vi "change pivot.vi"(6 "force recalc?":bool, 7 "Use bumper corners?":bool=TRUE, 8 "error in (no error)":errorcluster, 9 "new pivot center":T1 {"Y" format="%.4g"; "X" format="%.4g"}, 11 "select pivot point":T2) -> (0 "error out":errorcluster)   [LabVIEW 2023]
uses:
  ctrl defs/ctrl pivot select.ctl
  ctrl defs/ctrl XY coord.ctl
  ctrl defs/ctrl Wheel index.ctl
  Global odometry.vi
  Global INIT.vi
panel:
  in  "bumper (in)":dbl=3.5
  out "new pivot center 2":T1={"X"=-0.11812379110251395, "Y"=-0.5906189555125736} {"Y" format="%.4g"; "X" format="%.4g"}
  out "recalc mod polar":bool=TRUE
  out "output pivot center":T1={"X"=-0.11812379110251395, "Y"=-0.5906189555125736} {"Y" format="%.4g"; "X" format="%.4g"}
  out "Old pivot center":T1 {"Y" format="%.4g"; "X" format="%.4g"}
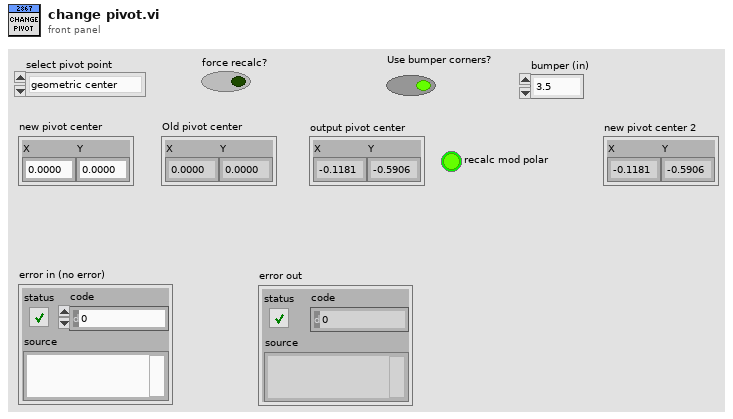
[diagram p1: front panel]
types:
  T1 = typedef "ctrl XY coord.ctl" = cluster{"X":dbl, "Y":dbl}
  T2 = typedef "ctrl pivot select.ctl" = enum16{"geometric center", "CG", "FL", "FR", "RR", "RL", "other"}
  T3 = typedef "ctrl robot swerve dims.ctl" = cluster{"width":dbl, "depth":dbl}
  T4 = cluster{"description":string, "wrt geom CTR":cluster{"delX":i8, "delY":i8}}[]
  T5 = typedef "ctrl swerve module.ctl" = cluster{"descr":string, "V":dbl, "POS":dbl, "target":dbl, "ABS":dbl, "from pivot to module":cluster{"R":dbl, "theta (deg)":dbl, "theta spin (deg)":dbl, "theta park (deg)":dbl}, "coord wrt geom CTR":cluster{"X":dbl, "Y":dbl}, "corner wt (lbm)":dbl}
  T6 = typedef "ctrl robot CG.ctl" = cluster{"mass (lbm)":dbl, "CG":T1, "Zcg":dbl}
  T7 = typedef "ctrl Wheel index.ctl" = enum16{"FR", "FL", "RL", "RR"}
  T8 = cluster{"description":string, "wrt geom CTR":cluster{"delX":i8, "delY":i8}}
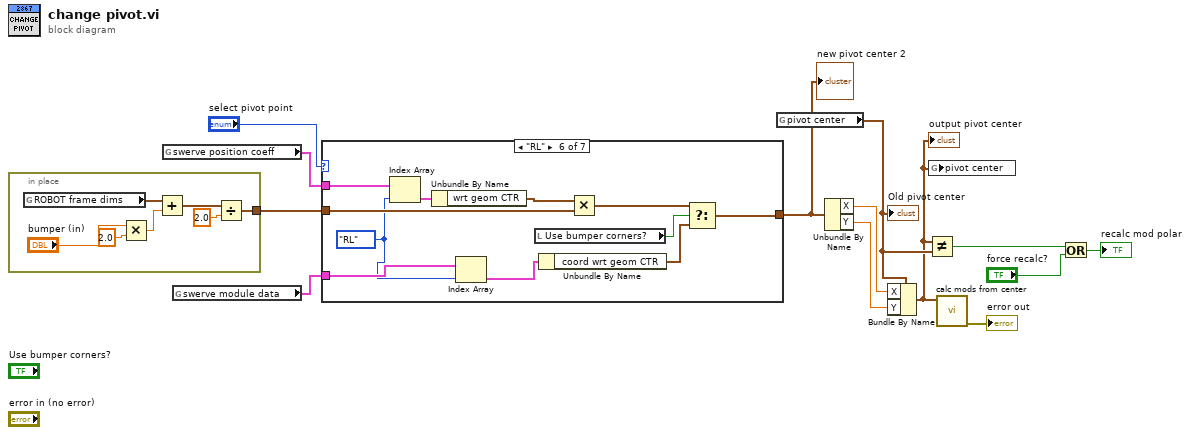
[diagram p0: block diagram]
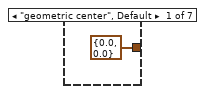
[diagram p2: hidden frame]
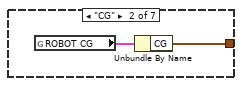
[diagram p3: hidden frame]
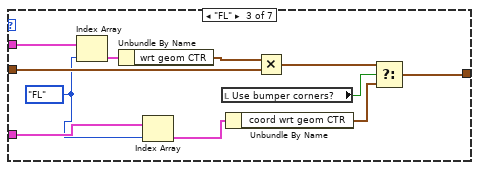
[diagram p4: hidden frame]
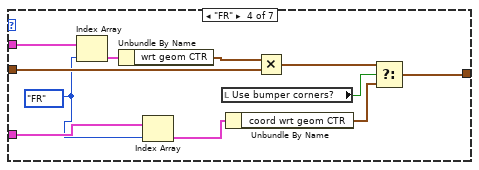
[diagram p5: hidden frame]
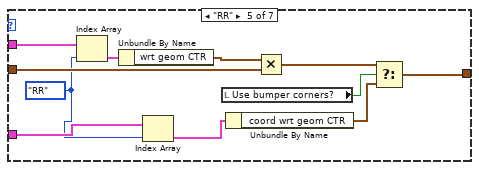
[diagram p6: hidden frame]
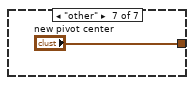
[diagram p7: hidden frame]
diagram:
  n1 = in-place {
    in-place-border: [w15] -> w2
    n2 = global read "Global INIT.vi" "ROBOT frame dims"() -> (w20:T3)
    n3 = Multiply(x="bumper (in)", y=2.0) -> (x*y=w19:dbl)
    n4 = Add(x=w20, y=w19) -> (x+y=w16:T3)
    n5 = Divide(x=w16, y=2.0) -> (x/y=w15:T3)
  }
  n6 = global read "Global INIT.vi" "swerve position coeff"() -> (w1:T4)
  n7 = global read "Global odometry.vi" "swerve module data"() -> (w12:T5[])
  n8 = case shown="\"RL\"" "select pivot point" {
    tunnel: [T1 {"X"=0.0, "Y"=0.0} ("CG") w22 w28 w39 w50 w61 "new pivot center"] -> w7
    tunnel: w12 -> [_ _ w34 w45 w56 w67 _]
    tunnel: w2 -> [_ _ w29 w40 w51 w62 _]
    tunnel: w1 -> [_ _ w32 w43 w54 w65 _]
    frame "geometric center", Default {
    }
    frame "CG" {
      n9 = global read "Global INIT.vi" "ROBOT CG"() -> (w23:T6)
      n10 = Unbundle By Name(w23) -> ("CG"=w22:T1)
    }
    frame "FL" {
      w24 = ctrl_Wheel_index."FL" ("Wheel index")
      n11 = Index Array(array=w32, index=w24) -> (element=w31:T8)
      n12 = Unbundle By Name(w31) -> ("wrt geom CTR"=w30:cluster{"delX":i8, "delY":i8})
      n13 = Index Array(array=w34, index=w24) -> (element=w33:T5)
      n14 = local read "Use bumper corners?"() -> (w25:bool)
      n15 = Unbundle By Name(w33) -> ("coord wrt geom CTR"=w26:cluster{"X":dbl, "Y":dbl})
      n16 = Multiply(x=w30, y=w29) -> (x*y=w27:T3)
      n17 = Select(t=w27, s=w25, f=w26) -> (s? t:f=w28:T3)
    }
    frame "FR" {
      w35 = ctrl_Wheel_index."FR" ("Wheel index")
      n18 = Index Array(array=w43, index=w35) -> (element=w42:T8)
      n19 = Unbundle By Name(w42) -> ("wrt geom CTR"=w41:cluster{"delX":i8, "delY":i8})
      n20 = Index Array(array=w45, index=w35) -> (element=w44:T5)
      n21 = local read "Use bumper corners?"() -> (w36:bool)
      n22 = Unbundle By Name(w44) -> ("coord wrt geom CTR"=w37:cluster{"X":dbl, "Y":dbl})
      n23 = Multiply(x=w41, y=w40) -> (x*y=w38:T3)
      n24 = Select(t=w38, s=w36, f=w37) -> (s? t:f=w39:T3)
    }
    frame "RR" {
      w46 = ctrl_Wheel_index."RR" ("Wheel index")
      n25 = Index Array(array=w54, index=w46) -> (element=w53:T8)
      n26 = Unbundle By Name(w53) -> ("wrt geom CTR"=w52:cluster{"delX":i8, "delY":i8})
      n27 = Index Array(array=w56, index=w46) -> (element=w55:T5)
      n28 = local read "Use bumper corners?"() -> (w47:bool)
      n29 = Unbundle By Name(w55) -> ("coord wrt geom CTR"=w48:cluster{"X":dbl, "Y":dbl})
      n30 = Multiply(x=w52, y=w51) -> (x*y=w49:T3)
      n31 = Select(t=w49, s=w47, f=w48) -> (s? t:f=w50:T3)
    }
    frame "RL" {
      w57 = ctrl_Wheel_index."RL" ("Wheel index")
      n32 = Index Array(array=w65, index=w57) -> (element=w64:T8)
      n33 = Unbundle By Name(w64) -> ("wrt geom CTR"=w63:cluster{"delX":i8, "delY":i8})
      n34 = Index Array(array=w67, index=w57) -> (element=w66:T5)
      n35 = local read "Use bumper corners?"() -> (w58:bool)
      n36 = Unbundle By Name(w66) -> ("coord wrt geom CTR"=w59:cluster{"X":dbl, "Y":dbl})
      n37 = Multiply(x=w63, y=w62) -> (x*y=w60:T3)
      n38 = Select(t=w60, s=w58, f=w59) -> (s? t:f=w61:T3)
    }
    frame "other" {
    }
  }
  "new pivot center 2" <- w7
  n39 = global read "Global odometry.vi" "pivot center"() -> (w10:T1)
  "Old pivot center" <- w10
  n40 = Unbundle By Name(w7) -> ("X"=w9:dbl, "Y"=w8:dbl)
  n41 = Bundle By Name(cluster=w10, "X"=w9, "Y"=w8) -> (w3:T1)
  "output pivot center" <- w3
  n42 = Not Equal?(x=w3, y=w10) -> (x != y?=w11:bool)
  n43 = global write "Global odometry.vi" "pivot center"(w3) -> ()
  n44 = call "calc mods from center.vi"("pivot center"=w3) -> ("error out"=→"error out":errorcluster)  [unwired: 10 in]
  n45 = Or(x=w11, y="force recalc?") -> (x .or. y?=→"recalc mod polar":bool)
